vi "subtractVectors.vi"(8 "y2":dbl, 9 "x2":dbl, 10 "y1":dbl, 11 "x1":dbl) -> (1 "y":dbl, 2 "x":dbl)   [LabVIEW 2016]
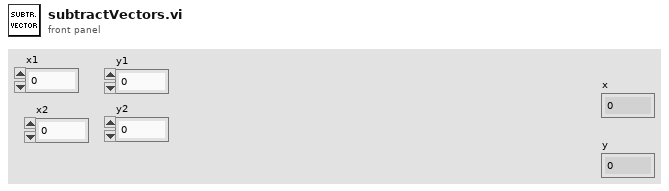
[diagram p1: front panel]
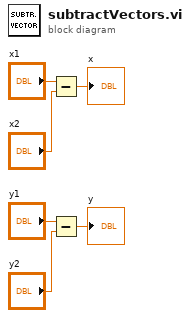
[diagram p0: block diagram]
diagram:
  n1 = Subtract(x="x1", y="x2") -> (x-y=→"x":dbl)
  n2 = Subtract(x="y1", y="y2") -> (x-y=→"y":dbl)
